vi "稱號-骰子賭爛.vi"() -> ()   [LabVIEW 2014]
panel:
  in  "退出視窗":bool
  # "恭喜獲得稱號:"
  # "代表你在骰子方面的賭運非常不好，奉勸你現實中千萬\n不要玩跟骰子有關的賭博，會輸很慘的。"
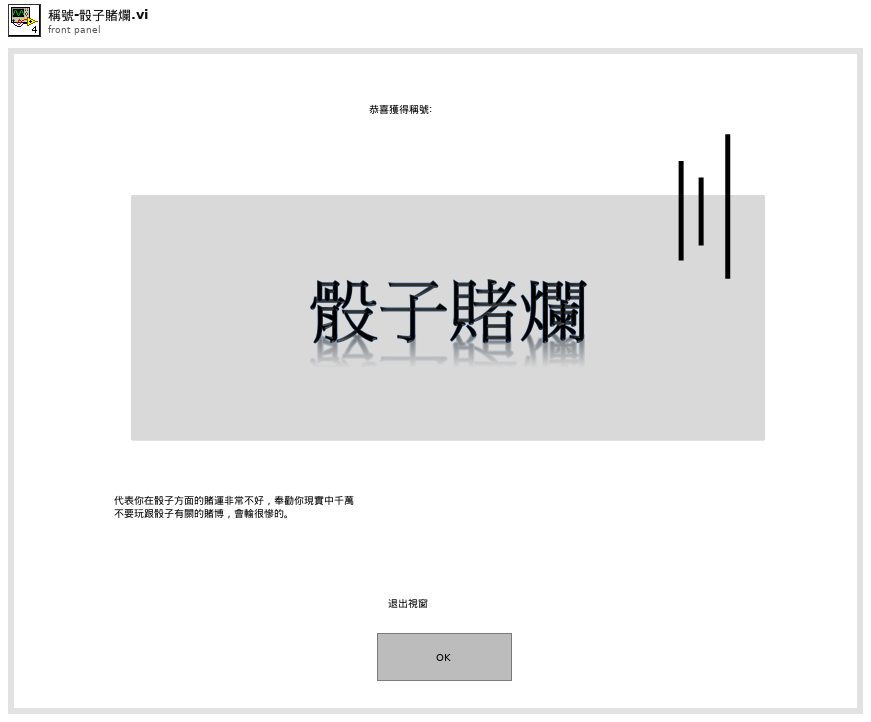
[diagram p1: front panel]
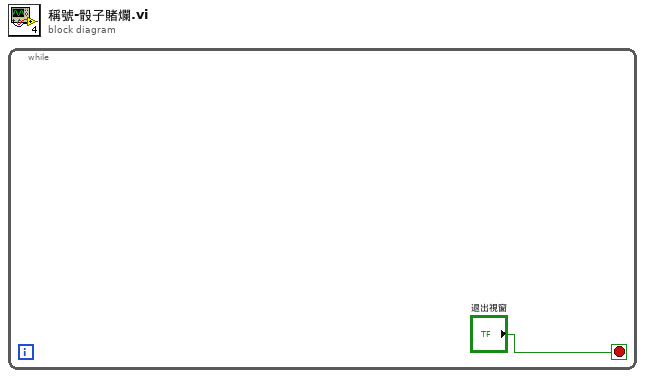
[diagram p0: block diagram]
diagram:
  n1 = while {
    stop <- "退出視窗" stop-if-true
  }
